vi "Calculate Setpoint.vi"(8 "error in (no error)":errorcluster, 10 "time (sec)":dbl, 11 "Parabolic Setpoint in":refnum<class "Parabolic Setpoint.lvclass">) -> (0 "error out":errorcluster, 1 "type":string, 2 "setpoint":dbl, 3 "Parabolic Setpoint out":refnum<class "Parabolic Setpoint.lvclass">, 5 "testing?":bool)   [LabVIEW 2020, in "Parabolic Setpoint.lvclass"]
uses:
  Parabolic Setpoint.lvclass
  C:/Users/jason/Documents/Inflation-Apparatus/src/Inflation Test/Parameter Class/IA Test Parameters.lvclass
  Parabolic Setpoint.lvclass/Parabolic Setpoint.ctl
  IA Test Parameters.lvclass/IA Test Parameters.ctl
  IA Test Parameters.lvclass
  C:/Users/jason/Documents/Inflation-Apparatus/src/Inflation Test/Parameter Class/Setpoints/Parabolic Setpoint/Parabolic Setpoint.lvclass
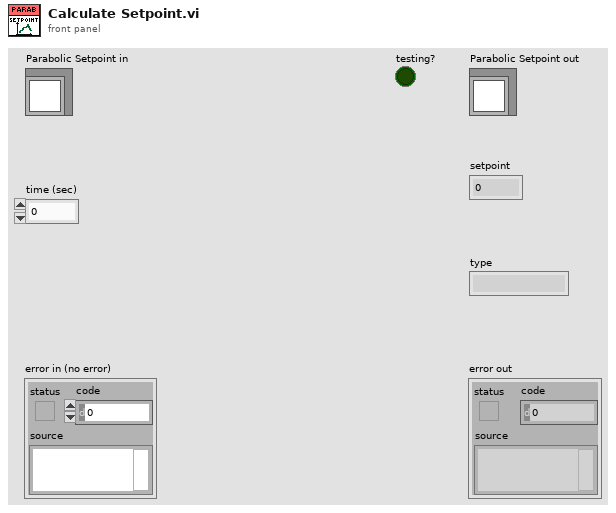
[diagram p1: front panel]
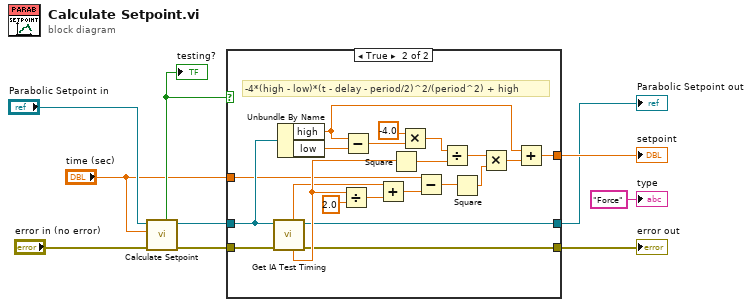
[diagram p0: block diagram]
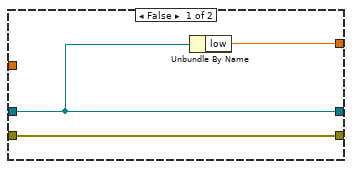
[diagram p2: hidden frame]
diagram:
  n1 = call-parent "Calculate Setpoint.vi"("error in (no error)"="error in (no error)", "time (sec)"="time (sec)", "IA Test Parameters in"="Parabolic Setpoint in") -> ("error out"=w8:errorcluster, "IA Test Parameters out"=w7:refnum<class "Parabolic Setpoint.lvclass">, "testing?"=w6:bool)  [unwired: 4 in, 2 out]
  "testing?" <- w6
  n2 = case shown="True" w6 {
    tunnel: w8 -> [w12 w34]
    tunnel: w7 -> [w11 w33]
    tunnel: "time (sec)" -> [_ w23]
    tunnel: [w13 w19] -> w4
    tunnel: [w12 w17] -> w3
    tunnel: [w11 w18] -> w1
    frame False {
      n3 = Unbundle By Name(w11) -> ("low"=w13:dbl)
    }
    frame True {
      # "-4*(high - low)*(t - delay - period/2)^2/(period^2) + high"
      n4 = call "Get IA Test Timing.vi"("error in (no error)"=w34, "IA Test Parameters in"=w33) -> ("error out"=w17:errorcluster, "IA Test Parameters out"=w18:refnum<class "Parabolic Setpoint.lvclass">, "test period (sec)"=w27:dbl, "time delay (sec)"=w24:dbl)  [unwired: 4 in, 2 out]
      n5 = Unbundle By Name(w33) -> ("high"=w21:dbl, "low"=w32:dbl)
      n6 = Divide(x=w27, y=2.0) -> (x/y=w25:dbl)
      n7 = Subtract(x=w21, y=w32) -> (x-y=w31:dbl)
      n8 = Add(x=w24, y=w25) -> (x+y=w22:dbl)
      n9 = Square(x=w27) -> (x^2=w28:dbl)
      n10 = Multiply(x=-4.0, y=w31) -> (x*y=w29:dbl)
      n11 = Subtract(x=w23, y=w22) -> (x-y=w16:dbl)
      n12 = Divide(x=w29, y=w28) -> (x/y=w14:dbl)
      n13 = Square(x=w16) -> (x^2=w15:dbl)
      n14 = Multiply(x=w14, y=w15) -> (x*y=w20:dbl)
      n15 = Add(x=w21, y=w20) -> (x+y=w19:dbl)
    }
  }
  "error out" <- w3
  "Parabolic Setpoint out" <- w1
  "setpoint" <- w4
  "type" <- "Force" ("type")
